vi "Generate_Map.vi"(4 "current position":dbl[](array[numeric]), 6 "corner 2":dbl[](array[numeric]), 7 "2D array":dbl[][](array[numeric]), 8 "corner 1":dbl[](array[numeric]), 9 "POV":bool, 10 "Map M1(t)/M2(f)":bool, 11 "Display Corner Positions?":bool) -> (0 "Cluster Array Plot":cluster{dbl[], dbl[]}[](array[cluster]), 2 "POV":bool)   [LabVIEW 2018]
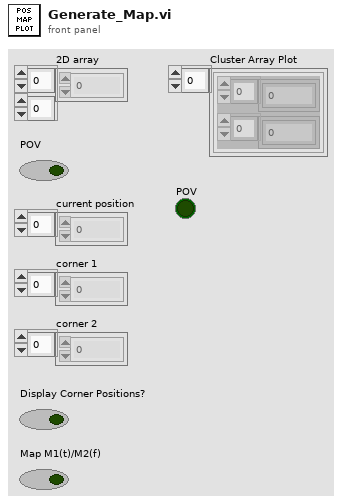
[diagram p1: front panel]
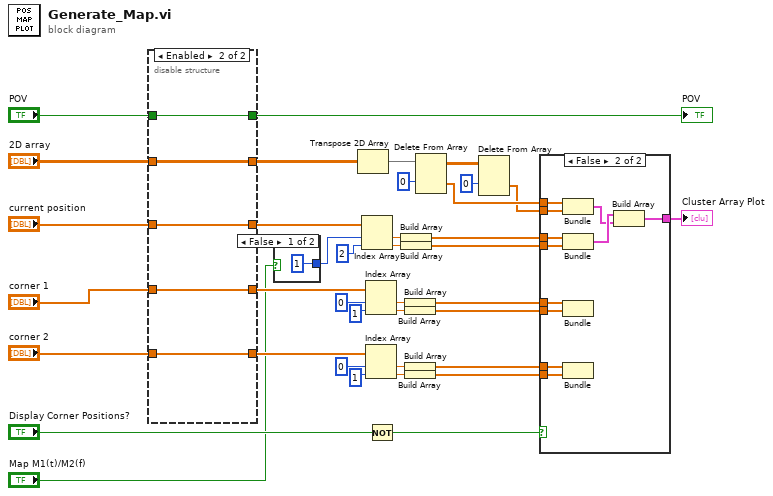
[diagram p0: block diagram]
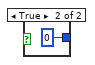
[diagram p2: hidden frame]
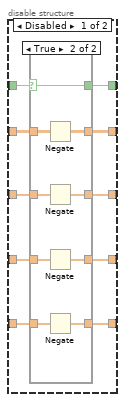
[diagram p3: hidden frame]
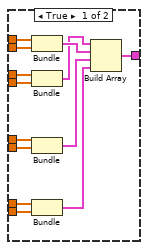
[diagram p5: hidden frame]
diagram:
  n1 = disable-structure shown="Enabled" {
    disable-tunnel: "2D array" -> [w48 w67]
    disable-tunnel: [w47 w67] -> w31
    disable-tunnel: "POV" -> [w46 w63]
    disable-tunnel: "current position" -> [w45 w66]
    disable-tunnel: [w44 w66] -> w9
    disable-tunnel: "corner 1" -> [w43 w65]
    disable-tunnel: "corner 2" -> [w42 w64]
    disable-tunnel: [w41 w65] -> w6
    disable-tunnel: [w40 w64] -> w5
    disable-tunnel: [w39 w63] -> w4
    frame Disabled {
      n2 = case shown="True" w46 {
        selector: w46 -> [w49 w54]
        tunnel: w48 -> [w53 w62]
        tunnel: [w53 w61] -> w47
        tunnel: w45 -> [w52 w60]
        tunnel: [w52 w59] -> w44
        tunnel: w43 -> [w51 w58]
        tunnel: w42 -> [w50 w57]
        tunnel: [w51 w56] -> w41
        tunnel: [w50 w55] -> w40
        tunnel: [w49 w54] -> w39
        frame False {
        }
        frame True {
          n3 = Negate(x=w62) -> (-x=w61:dbl[][])
          n4 = Negate(x=w60) -> (-x=w59:dbl[])
          n5 = Negate(x=w58) -> (-x=w56:dbl[])
          n6 = Negate(x=w57) -> (-x=w55:dbl[])
        }
      }
    }
    frame Enabled {
    }
  }
  "POV" <- w4
  n7 = case shown="False" "Map M1(t)/M2(f)" {
    tunnel: [1 ("index") 0 ("index")] -> w1
    frame False {
    }
    frame True {
    }
  }
  n8 = Transpose 2D Array(2D array=w31) -> (transposed array=w33:dbl[][])
  n9 = Index Array(array=w9, index #1=w1, index #2=2 ("index")) -> (element #1=w29:dbl, element #2=w28:dbl)
  n10 = Index Array(array=w6, index #1=0 ("index"), index #2=1 ("index")) -> (element #1=w24:dbl, element #2=w25:dbl)
  n11 = Index Array(array=w5, index #1=0 ("index"), index #2=1 ("index")) -> (element #1=w19:dbl, element #2=w18:dbl)
  n12 = Not(x="Display Corner Positions?") -> (.not. x?=w11:bool)
  n13 = Build Array(w29) -> (w27:dbl[])
  n14 = Build Array(w28) -> (w26:dbl[])
  n15 = Build Array(w24) -> (w17:dbl[])
  n16 = Build Array(w25) -> (w16:dbl[])
  n17 = Build Array(w19) -> (w15:dbl[])
  n18 = Build Array(w18) -> (w14:dbl[])
  n19 = Delete From Array(array=w33, index (row)=0) -> (deleted portion=w35:dbl[], array with subset deleted=w37:dbl[][])  [unwired: 2 in]
  n20 = Delete From Array(array=w37, index (row)=0) -> (deleted portion=w34:dbl[])  [unwired: 2 in, 1 out]
  n21 = case shown="False" w11 {
    tunnel: w35 -> [w82 w93]
    tunnel: w34 -> [w81 w92]
    tunnel: w27 -> [w80 w91]
    tunnel: w26 -> [w79 w90]
    tunnel: w17 -> [w78 w89]
    tunnel: w16 -> [w77 w88]
    tunnel: w15 -> [w76 w87]
    tunnel: w14 -> [w75 w86]
    tunnel: [w72 w85] -> w13
    frame True {
      n22 = Bundle(w82, w81) -> (w71:cluster{dbl[], dbl[]})  [unwired: 1 in]
      n23 = Bundle(w80, w79) -> (w70:cluster{dbl[], dbl[]})  [unwired: 1 in]
      n24 = Bundle(w78, w77) -> (w74:cluster{dbl[], dbl[]})  [unwired: 1 in]
      n25 = Bundle(w76, w75) -> (w73:cluster{dbl[], dbl[]})  [unwired: 1 in]
      n26 = Build Array(w70, w71, w74, w73) -> (w72:cluster{dbl[], dbl[]}[])
    }
    frame False {
      n27 = Bundle(w93, w92) -> (w83:cluster{dbl[], dbl[]})  [unwired: 1 in]
      n28 = Bundle(w91, w90) -> (w84:cluster{dbl[], dbl[]})  [unwired: 1 in]
      n29 = Bundle(w89, w88) -> ()  [unwired: 1 in, 1 out]
      n30 = Bundle(w87, w86) -> ()  [unwired: 1 in, 1 out]
      n31 = Build Array(w84, w83) -> (w85:cluster{dbl[], dbl[]}[])
    }
  }
  "Cluster Array Plot" <- w13
